vi "User Front Panel.vi"(8 "PanelCMDRef":refnum<vi>, 11 "PanelCluster":T6) -> ()   [LabVIEW 2019]
uses:
  <vilib>/Native 3D Graph/xcontrol/3DPC_SurfacePlot.xctl
  CoreModules/StationModule/StationData.ctl
panel:
  in  "Tab Control":enum32{"User", "Parameter"}(tab)
  out "PathPlot":refnum<class "Base Datatype.lvclass">[](xcontrol)
  in  "Test":bool
  in  "test123":bool
  in  "ID1":bool
  in  "ID2":bool
  in  "ID3":bool
  in  "ID4":bool
  in  "ID5":bool
  in  "ID6":bool
  in  "ID7":bool
  in  "ID8":bool
  in  "ID9":bool
  in  "ID10":bool
  in  "ID12":bool
  in  "ID11":bool
  in  "LensBuffer":T1
  in  "VcmBuffer":cluster{"1":bool, "2":bool, "3":bool, "4":bool}
  in  "testtray":T2
  out "appended path":path
  in  "FeedIn":T3
  in  "FeedOut":T4
  out "Image":T5(plugin-control)
  out "Waveform":waveform(dbl)[](graph)
  in  "CRDCMPT4Y":string
  in  "CRDCMPT4X":string
  in  "CRDCMPT4Org":string
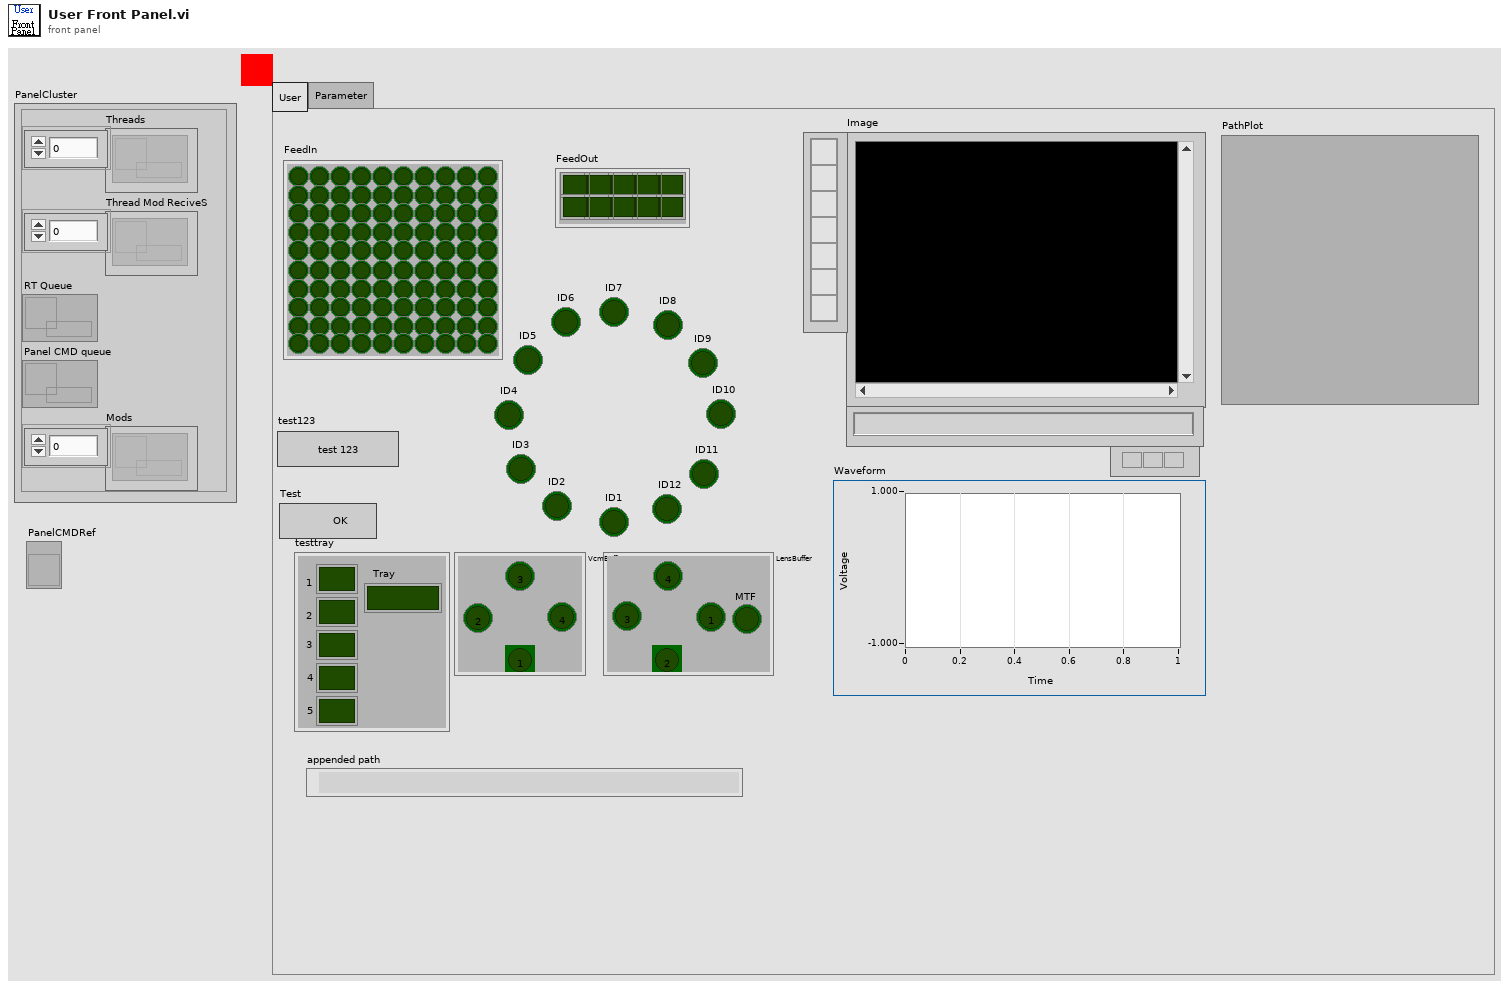
[diagram p1: front panel]
types:
  T1 = cluster{"MTF":bool, "1":bool, "2":bool, "3":bool, "4":bool}
  T2 = cluster{"Tray":bool, "1":bool, "2":bool, "3":bool, "4":bool, "5":bool}
  T3 = cluster{"1":bool, "2":bool, "3":bool, "4":bool, "5":bool, "6":bool, "7":bool, "8":bool, "9":bool, "10":bool, "1 2":bool, "2 2":bool, "3 2":bool, "4 2":bool, "5 2":bool, "6 2":bool, "7 2":bool, "8 2":bool, "9 2":bool, "10 2":bool, "1 3":bool, "2 3":bool, "3 3":bool, "4 3":bool, "5 3":bool, "6 3":bool, "7 3":bool, "8 3":bool, "9 3":bool, "10 3":bool, "1 4":bool, "2 4":bool, "3 4":bool, "4 4":bool, "5 4":bool, "6 4":bool, "7 4":bool, "8 4":bool, "9 4":bool, "10 4":bool, "1 5":bool, "2 5":bool, "3 5":bool, "4 5":bool, "5 5":bool, "6 5":bool, "7 5":bool, "8 5":bool, "9 5":bool, "10 5":bool, "1 6":bool, "2 6":bool, "3 6":bool, "4 6":bool, "5 6":bool, "6 6":bool, "7 6":bool, "8 6":bool, "9 6":bool, "10 6":bool, "1 7":bool, "2 7":bool, "3 7":bool, "4 7":bool, "5 7":bool, "6 7":bool, "7 7":bool, "8 7":bool, "9 7":bool, "10 7":bool, "1 8":bool, "2 8":bool, "3 8":bool, "4 8":bool, "5 8":bool, "6 8":bool, "7 8":bool, "8 8":bool, "9 8":bool, "10 8":bool, "1 9":bool, "2 9":bool, "3 9":bool, "4 9":bool, "5 9":bool, "6 9":bool, "7 9":bool, "8 9":bool, "9 9":bool, "10 9":bool, "1 10":bool, "2 10":bool, "3 10":bool, "4 10":bool, "5 10":bool, "6 10":bool, "7 10":bool, "8 10":bool, "9 10":bool, "10 10":bool}
  T4 = cluster{"1":bool, "2":bool, "3":bool, "4":bool, "5":bool, "1 2":bool, "2 2":bool, "3 2":bool, "4 2":bool, "5 2":bool}
  T5 = typedef "IMAQ Image.ctl" = refnum<image>
  T6 = cluster{"Threads":refnum<queue>[], "Thread Mod ReciveS":refnum<queue>[], "RT Queue":refnum<queue>, "Panel CMD queue":refnum<queue>, "Mods":refnum<queue>[]}
  T7 = typedef "StationData.ctl" = enum16{"ResetDefault", "SetStationOK", "SetStationNG", "UpdateIndicator", "GetData", "SetData", "StateShift", "Init", "SetStationON", "SetStationOFF", "BlinkingON", "BlinkingOFF"}
  T8 = enum16{"Init", "AddStation", "StateShift", "ResetDefault", "SetStationON", "SetStationOFF", "SetStationOK", "SetStationNG", "UpdateIndicator", "SetData", "GetData", "GetOnOff", "GetOkNg"}
  T9 = cluster{"Program":i32, "Prog Index":i32, "State Index":i32, "State":enum16{"Init", "Idle", "Auto Start", "Auto Running", "Step Start", "Step Running", "Suspend", "Restart", "Stop", "Reset"}}
  T10 = enum16{"Get", "UpdatePointS", "Init", "UpdateIndex", "GetCurrent&Index+1", "GetWithIndex", "ChkLast", "GetCurrent"}
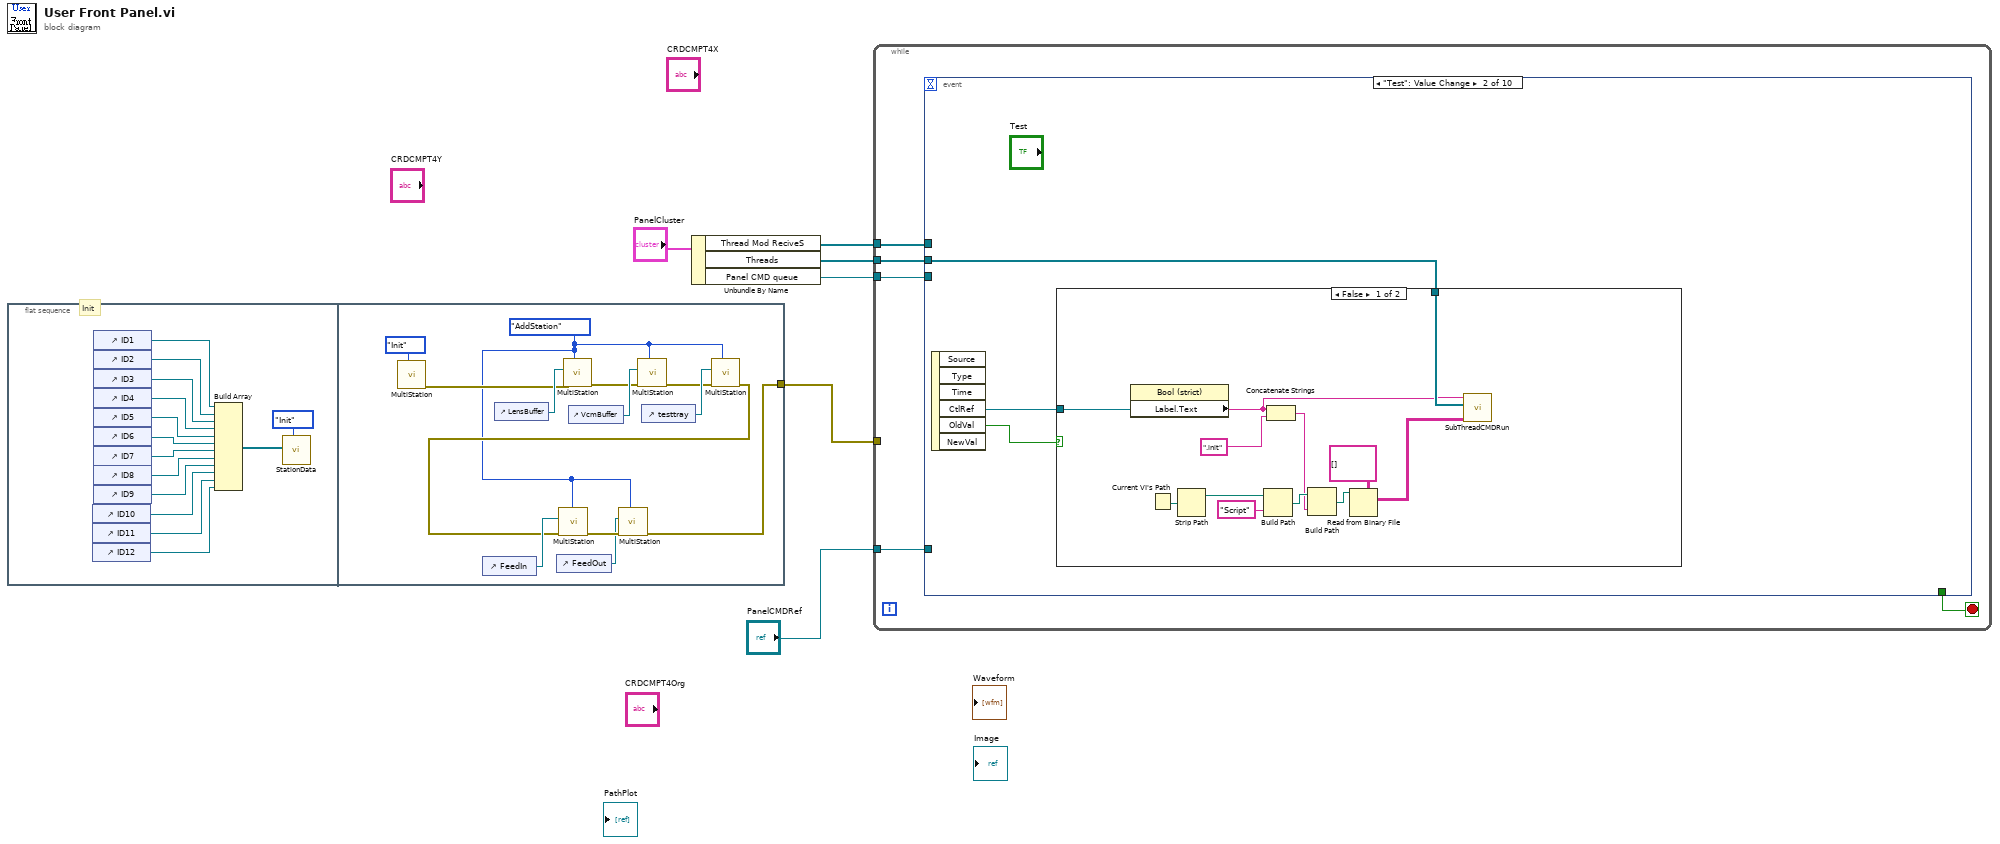
[diagram p0: block diagram]
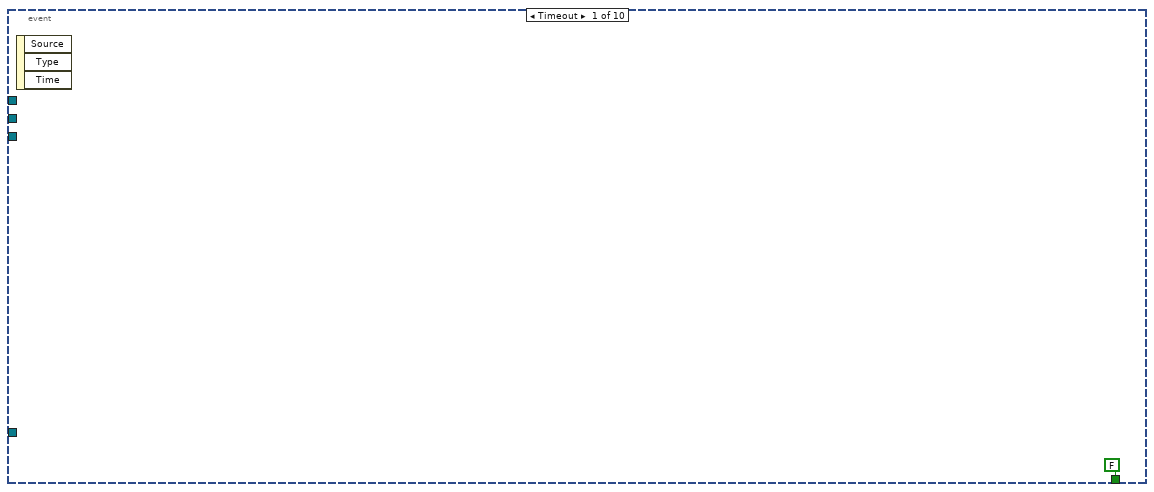
[diagram p2: hidden frame]
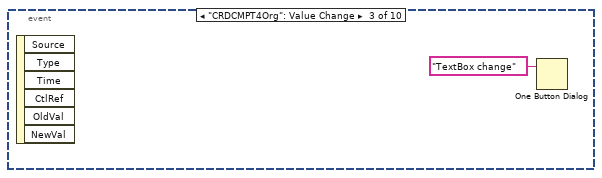
[diagram p4: hidden frame]
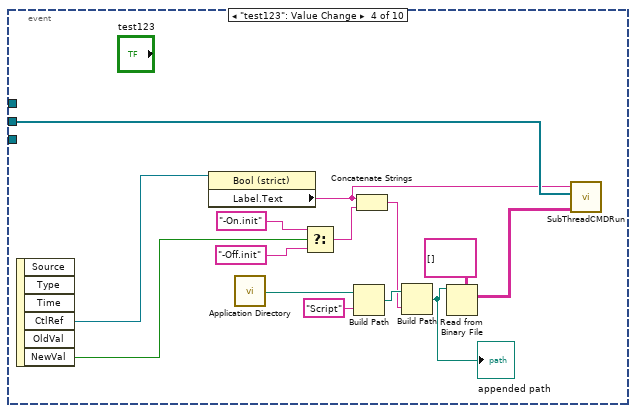
[diagram p5: hidden frame]
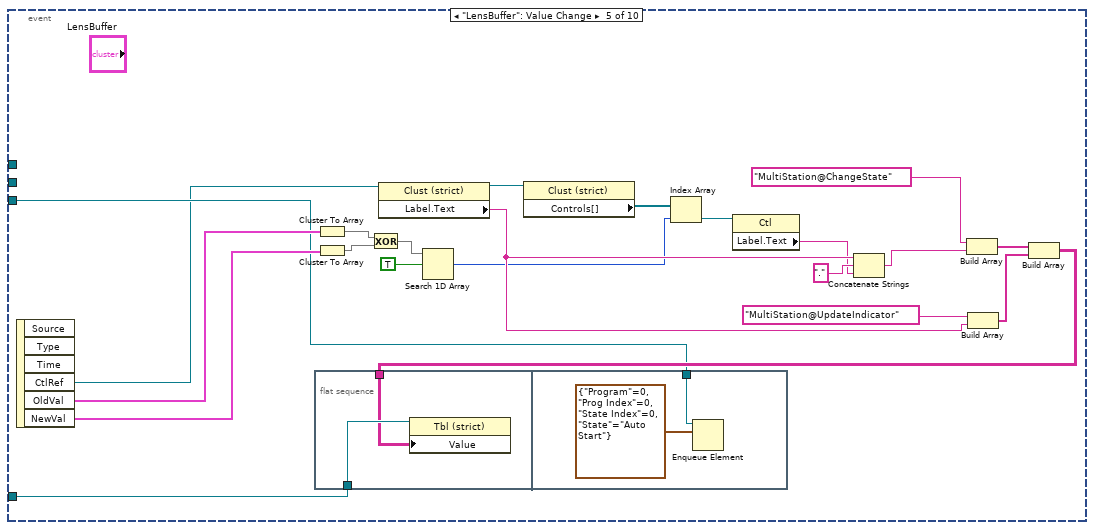
[diagram p6: hidden frame]
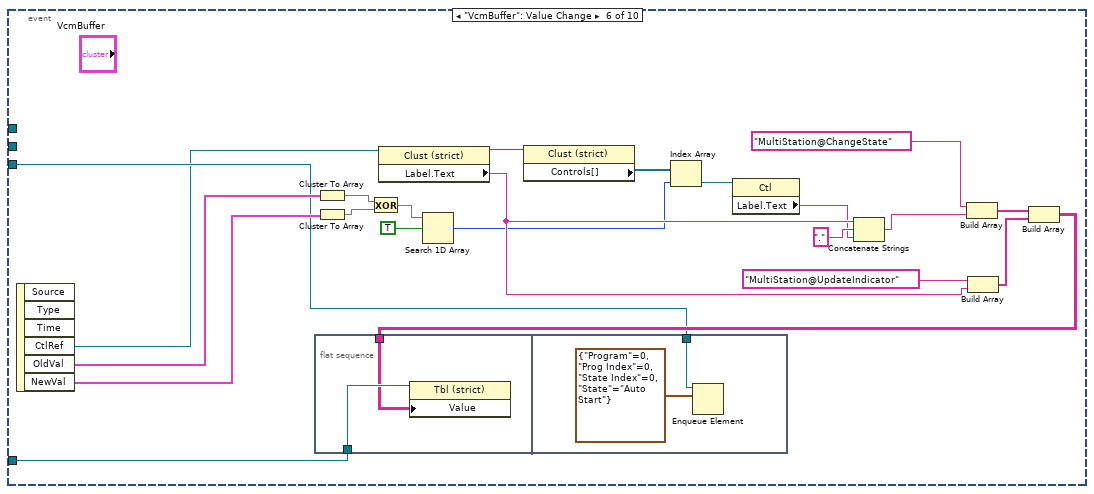
[diagram p7: hidden frame]
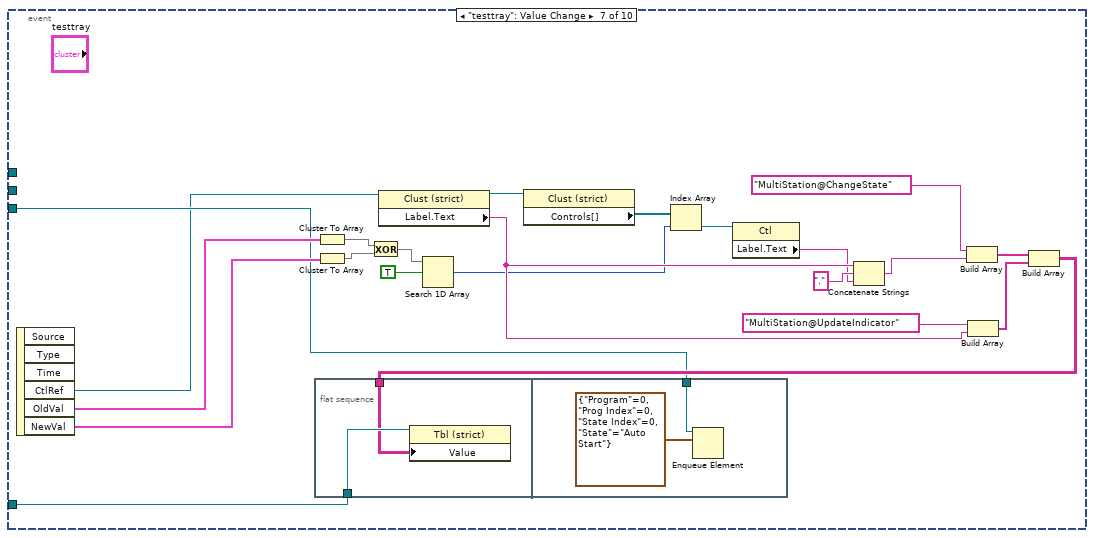
[diagram p8: hidden frame]
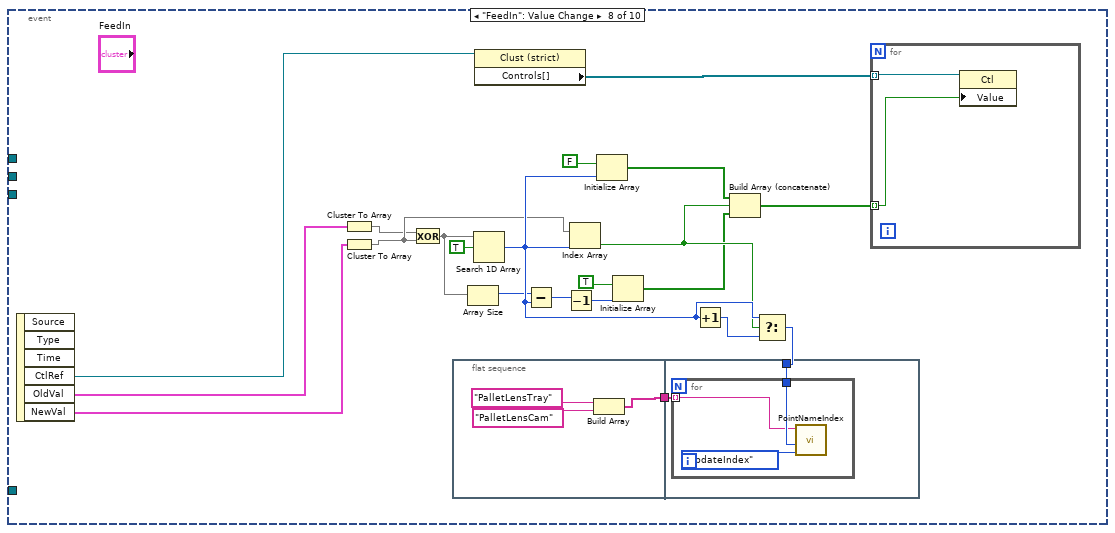
[diagram p9: hidden frame]
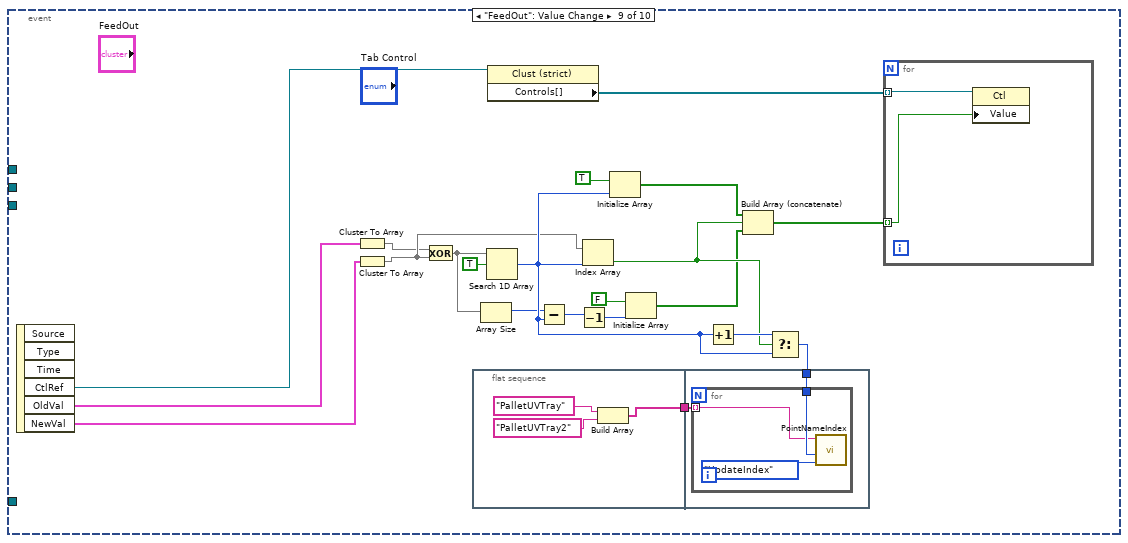
[diagram p10: hidden frame]
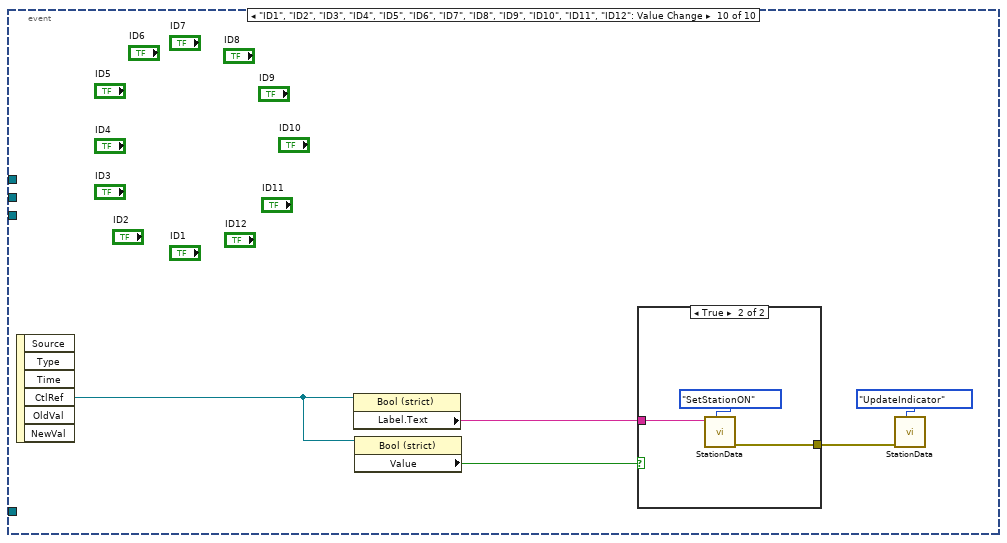
[diagram p11: hidden frame]
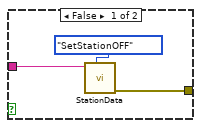
[diagram p12: hidden frame]
diagram:
  # "Init"
  n1 = flat-sequence {
    tunnel: [w22] -> w2
    frame #0 {
      n2 = control-ref of="ID10"() -> (w16:refnum<vi>)
      n3 = control-ref of="ID11"() -> (w17:refnum<vi>)
      n4 = control-ref of="ID12"() -> (w18:refnum<vi>)
      n5 = control-ref of="ID1"() -> (w7:refnum<vi>)
      n6 = control-ref of="ID2"() -> (w8:refnum<vi>)
      n7 = control-ref of="ID3"() -> (w9:refnum<vi>)
      n8 = control-ref of="ID4"() -> (w10:refnum<vi>)
      n9 = control-ref of="ID5"() -> (w11:refnum<vi>)
      n10 = control-ref of="ID6"() -> (w12:refnum<vi>)
      n11 = control-ref of="ID7"() -> (w13:refnum<vi>)
      n12 = control-ref of="ID8"() -> (w14:refnum<vi>)
      n13 = control-ref of="ID9"() -> (w15:refnum<vi>)
      n14 = Build Array(w7, w8, w9, w10, w11, w12, w13, w14, w15, w16, w17, w18) -> (w20:refnum<vi>[])
      n15 = call "StationData.vi"("CMD"=StationData."Init", "variant"=w20) -> ()  [unwired: 2 in, 8 out]
    }
    frame #1 {
      w23 = T8."AddStation" ("OP")
      n16 = call "MultiStation.vi"("OP"=T8."Init") -> ("error out"=w27:errorcluster)  [unwired: 6 in, 4 out]
      n17 = control-ref of="FeedIn"() -> (w26:refnum<vi>)
      n18 = control-ref of="LensBuffer"() -> (w33:refnum<vi>)
      n19 = control-ref of="FeedOut"() -> (w21:refnum<vi>)
      n20 = call "MultiStation.vi"("OP"=w23, "error in"=w27, "DataIn"=w33) -> ("error out"=w30:errorcluster)  [unwired: 4 in, 4 out]
      n21 = control-ref of="VcmBuffer"() -> (w32:refnum<vi>)
      n22 = call "MultiStation.vi"("OP"=w23, "error in"=w30, "DataIn"=w32) -> ("error out"=w29:errorcluster)  [unwired: 4 in, 4 out]
      n23 = control-ref of="testtray"() -> (w31:refnum<vi>)
      n24 = call "MultiStation.vi"("OP"=w23, "error in"=w29, "DataIn"=w31) -> ("error out"=w25:errorcluster)  [unwired: 4 in, 4 out]
      n25 = call "MultiStation.vi"("OP"=w23, "error in"=w25, "DataIn"=w26) -> ("error out"=w24:errorcluster)  [unwired: 4 in, 4 out]
      n26 = call "MultiStation.vi"("OP"=w23, "error in"=w24, "DataIn"=w21) -> ("error out"=w22:errorcluster)  [unwired: 4 in, 4 out]
    }
  }
  n27 = Unbundle By Name("PanelCluster") -> ("Thread Mod ReciveS"=w5:refnum<queue>[], "Threads"=w4:refnum<queue>[], "Panel CMD queue"=w3:refnum<queue>)
  n28 = while {
    tunnel: w5 -> [w36]
    tunnel: w4 -> [w37]
    tunnel: w3 -> [w35]
    tunnel: w2 -> [_]
    tunnel: "PanelCMDRef" -> [w34]
    stop <- w38 stop-if-true
    n29 = event shown="[1] \"Test\": Value Change" {
      selector: _ -> [_ _ _ _ _ _ _ _ _ _]
      dyn-events: _ -> [_ _ _ _ _ _ _ _ _ _]
      timeout: _ -> [_ _ _ _ _ _ _ _ _ _]
      tunnel: [FALSE _ _ _ _ _ _ _ _ _] -> w38
      tunnel: w37 -> [_ w42 _ w61 _ _ _ _ _ _]
      tunnel: w36 -> [_ _ _ _ _ _ _ _ _ _]
      tunnel: w35 -> [_ _ _ _ w72 w98 w124 _ _ _]
      tunnel: w34 -> [_ _ _ _ w70 w96 w122 _ _ _]
      event Timeout {
        n30 = event-data() -> ()  [unwired: 1 in, 3 out]
      }
      event "Test": Value Change {
        n31 = event-data() -> ("CtlRef"=w41:refnum<vi>, "OldVal"=w40:bool)  [unwired: 1 in, 4 out]
        n32 = case shown="False" w40 {
          tunnel: w42 -> [w54 _]
          tunnel: w41 -> [w53 _]
          frame False {
            n33 = property class="Bool (strict)"(reference=w53) -> ("Label.Text"=w43:string)  [unwired: 1 in, 2 out]
            n34 = Current VI's Path() -> (path=w47:path)
            n35 = Strip Path(path=w47) -> (stripped path=w46:path)  [unwired: 1 out]
            n36 = Build Path(base path=w46, name or relative path="Script") -> (appended path=w51:path)
            n37 = Concatenate Strings(w43, ".init" ("string")) -> (w50:string)
            n38 = Build Path(base path=w51, name or relative path=w50) -> (appended path=w49:path)
            n39 = Read from Binary File(5:string[][] [] ("Init Script"), 11:w49) -> (2:w45:string[][])  [unwired: 4 in, 3 out]
            n40 = call "SubThreadCMDRun.vi"("Command"=w45, "Threads"=w54, "SubThreadName"=w43) -> ()  [unwired: 8 in, 1 out]
          }
          frame True {
          }
        }
      }
      event "CRDCMPT4Org": Value Change {
        n41 = event-data() -> ()  [unwired: 1 in, 6 out]
        n42 = One Button Dialog(message="TextBox change") -> ()  [unwired: 1 in, 1 out]
      }
      event "test123": Value Change {
        n43 = event-data() -> ("CtlRef"=w60:refnum<vi>, "NewVal"=w59:bool)  [unwired: 1 in, 4 out]
        n44 = property class="Bool (strict)"(reference=w60) -> ("Label.Text"=w56:string)  [unwired: 1 in, 2 out]
        n45 = call <vilib>:"Application Directory.vi"() -> ("Application Directory"=w58:path)
        n46 = Select(t="-On.init", s=w59, f="-Off.init") -> (s? t:f=w65:string)
        n47 = Build Path(base path=w58, name or relative path="Script") -> (appended path=w68:path)
        n48 = Concatenate Strings(w56, w65) -> (w64:string)
        n49 = Build Path(base path=w68, name or relative path=w64) -> (appended path=w57:path)
        "appended path" <- w57
        n50 = Read from Binary File(5:string[][] [] ("Init Script"), 11:w57) -> (2:w62:string[][])  [unwired: 4 in, 3 out]
        n51 = call "SubThreadCMDRun.vi"("Command"=w62, "Threads"=w61, "SubThreadName"=w56) -> ()  [unwired: 8 in, 1 out]
      }
      event "LensBuffer": Value Change {
        n52 = event-data() -> ("CtlRef"=w71:refnum<vi>, "OldVal"=w74:T1, "NewVal"=w73:T1)  [unwired: 1 in, 3 out]
        n53 = flat-sequence {
          tunnel: w91 -> [w92]
          tunnel: w70 -> [w93]
          tunnel: w72 -> [w94]
          frame #0 {
            n54 = property class="Tbl (strict)"(reference=w93, "Value"=w92) -> ()  [unwired: 1 in, 2 out]
          }
          frame #1 {
            n55 = Enqueue Element(queue=w94, element=T9 {"Program"=0, "Prog Index"=0, "State Index"=0, "State"=enum."Auto Start"}) -> ()  [unwired: 1 in, 4 out]
          }
        }
        n56 = Cluster To Array(cluster=w74) -> (array=w75:bool[])
        n57 = Cluster To Array(cluster=w73) -> (array=w76:bool[])
        n58 = Exclusive Or(1:w76, 2:w75) -> (0:w77:bool[])
        n59 = property class="Clust (strict)"(reference=w71) -> (reference out=w79:refnum<vi>, "Label.Text"=w89:string)  [unwired: 1 in, 1 out]
        n60 = Search 1D Array(1D array=w77, element=TRUE) -> (index of element=w81:i32)  [unwired: 1 in]
        n61 = property class="Clust (strict)"(reference=w79) -> ("Controls[]"=w80:refnum<vi>[])  [unwired: 1 in, 2 out]
        n62 = Index Array(array=w80, index=w81) -> (element=w82:refnum<vi>)
        n63 = property class="Ctl"(reference=w82) -> ("Label.Text"=w83:string)  [unwired: 1 in, 2 out]
        n64 = Concatenate Strings(w89, "." ("string"), w83) -> (w86:string)
        n65 = Build Array("MultiStation@ChangeState", w86) -> (w87:string[])
        n66 = Build Array("MultiStation@UpdateIndicator", w89) -> (w90:string[])
        n67 = Build Array(w87, w90) -> (w91:string[][])
      }
      event "VcmBuffer": Value Change {
        n68 = event-data() -> ("CtlRef"=w97:refnum<vi>, "OldVal"=w100:cluster{"1":bool, "2":bool, "3":bool, "4":bool}, "NewVal"=w99:cluster{"1":bool, "2":bool, "3":bool, "4":bool})  [unwired: 1 in, 3 out]
        n69 = flat-sequence {
          tunnel: w117 -> [w118]
          tunnel: w96 -> [w119]
          tunnel: w98 -> [w120]
          frame #0 {
            n70 = property class="Tbl (strict)"(reference=w119, "Value"=w118) -> ()  [unwired: 1 in, 2 out]
          }
          frame #1 {
            n71 = Enqueue Element(queue=w120, element=T9 {"Program"=0, "Prog Index"=0, "State Index"=0, "State"=enum."Auto Start"}) -> ()  [unwired: 1 in, 4 out]
          }
        }
        n72 = Cluster To Array(cluster=w100) -> (array=w101:bool[])
        n73 = Cluster To Array(cluster=w99) -> (array=w102:bool[])
        n74 = Exclusive Or(1:w102, 2:w101) -> (0:w103:bool[])
        n75 = property class="Clust (strict)"(reference=w97) -> (reference out=w105:refnum<vi>, "Label.Text"=w115:string)  [unwired: 1 in, 1 out]
        n76 = Search 1D Array(1D array=w103, element=TRUE) -> (index of element=w107:i32)  [unwired: 1 in]
        n77 = property class="Clust (strict)"(reference=w105) -> ("Controls[]"=w106:refnum<vi>[])  [unwired: 1 in, 2 out]
        n78 = Index Array(array=w106, index=w107) -> (element=w108:refnum<vi>)
        n79 = property class="Ctl"(reference=w108) -> ("Label.Text"=w109:string)  [unwired: 1 in, 2 out]
        n80 = Concatenate Strings(w115, "." ("string"), w109) -> (w112:string)
        n81 = Build Array("MultiStation@ChangeState", w112) -> (w113:string[])
        n82 = Build Array("MultiStation@UpdateIndicator", w115) -> (w116:string[])
        n83 = Build Array(w113, w116) -> (w117:string[][])
      }
      event "testtray": Value Change {
        n84 = event-data() -> ("CtlRef"=w123:refnum<vi>, "OldVal"=w126:T2, "NewVal"=w125:T2)  [unwired: 1 in, 3 out]
        n85 = flat-sequence {
          tunnel: w143 -> [w144]
          tunnel: w122 -> [w145]
          tunnel: w124 -> [w146]
          frame #0 {
            n86 = property class="Tbl (strict)"(reference=w145, "Value"=w144) -> ()  [unwired: 1 in, 2 out]
          }
          frame #1 {
            n87 = Enqueue Element(queue=w146, element=T9 {"Program"=0, "Prog Index"=0, "State Index"=0, "State"=enum."Auto Start"}) -> ()  [unwired: 1 in, 4 out]
          }
        }
        n88 = Cluster To Array(cluster=w126) -> (array=w127:bool[])
        n89 = Cluster To Array(cluster=w125) -> (array=w128:bool[])
        n90 = Exclusive Or(1:w128, 2:w127) -> (0:w129:bool[])
        n91 = property class="Clust (strict)"(reference=w123) -> (reference out=w131:refnum<vi>, "Label.Text"=w141:string)  [unwired: 1 in, 1 out]
        n92 = Search 1D Array(1D array=w129, element=TRUE) -> (index of element=w133:i32)  [unwired: 1 in]
        n93 = property class="Clust (strict)"(reference=w131) -> ("Controls[]"=w132:refnum<vi>[])  [unwired: 1 in, 2 out]
        n94 = Index Array(array=w132, index=w133) -> (element=w134:refnum<vi>)
        n95 = property class="Ctl"(reference=w134) -> ("Label.Text"=w135:string)  [unwired: 1 in, 2 out]
        n96 = Concatenate Strings(w141, "." ("string"), w135) -> (w138:string)
        n97 = Build Array("MultiStation@ChangeState", w138) -> (w139:string[])
        n98 = Build Array("MultiStation@UpdateIndicator", w141) -> (w142:string[])
        n99 = Build Array(w139, w142) -> (w143:string[][])
      }
      event "FeedIn": Value Change {
        n100 = event-data() -> ("CtlRef"=w150:refnum<vi>, "OldVal"=w149:T3, "NewVal"=w148:T3)  [unwired: 1 in, 3 out]
        n101 = Cluster To Array(cluster=w149) -> (array=w151:bool[])
        n102 = Cluster To Array(cluster=w148) -> (array=w161:bool[])
        n103 = Exclusive Or(1:w161, 2:w151) -> (0:w154:bool[])
        n104 = flat-sequence {
          tunnel: [w169] -> w168
          tunnel: w165 -> [w173]
          tunnel: w168 -> [w172]
          frame #0 {
            n105 = Build Array("PalletLensTray", "PalletLensCam") -> (w169:string[])
          }
          frame #1 {
            n106 = for {
              tunnel: w173 -> [w176]
              tunnel: w172 -> [w175] mode=indexing
              n107 = call "PointNameIndex.vi"("OP"=T10."UpdateIndex", "PathIndexIn"=w176, "PointName"=w175) -> ()  [unwired: 3 in, 6 out]
            }
          }
        }
        n108 = Array Size(array=w154) -> (size(s)=w155:i32)
        n109 = Search 1D Array(1D array=w154, element=TRUE) -> (index of element=w167:i32)  [unwired: 1 in]
        n110 = property class="Clust (strict)"(reference=w150) -> ("Controls[]"=w162:refnum<vi>[])  [unwired: 1 in, 2 out]
        n111 = Subtract(x=w155, y=w167) -> (x-y=w159:i32)
        n112 = Decrement(x=w159) -> (x-1=w160:i32)
        n113 = Index Array(array=w161, index=w167) -> (element=w164:bool)
        n114 = Initialize Array(FALSE ("element"), w167) -> (w157:bool[])
        n115 = Initialize Array(TRUE ("element"), w160) -> (w158:bool[])
        n116 = Increment(x=w167) -> (x+1=w166:i32)
        n117 = Build Array (concatenate)(w157, w164, w158) -> (w163:bool[])
        n118 = Select(t=w167, s=w164, f=w166) -> (s? t:f=w165:i32)
        n119 = for {
          tunnel: w162 -> [w178] mode=indexing
          tunnel: w163 -> [w177] mode=indexing
          n120 = property class="Ctl"(reference=w178, "Value"=w177) -> ()  [unwired: 1 in, 2 out]
        }
      }
      event "FeedOut": Value Change {
        n121 = event-data() -> ("CtlRef"=w181:refnum<vi>, "OldVal"=w180:T4, "NewVal"=w179:T4)  [unwired: 1 in, 3 out]
        n122 = Cluster To Array(cluster=w180) -> (array=w182:bool[])
        n123 = Cluster To Array(cluster=w179) -> (array=w192:bool[])
        n124 = Exclusive Or(1:w192, 2:w182) -> (0:w185:bool[])
        n125 = flat-sequence {
          tunnel: [w200] -> w199
          tunnel: w196 -> [w204]
          tunnel: w199 -> [w203]
          frame #0 {
            n126 = Build Array("PalletUVTray", "PalletUVTray2") -> (w200:string[])
          }
          frame #1 {
            n127 = for {
              tunnel: w204 -> [w207]
              tunnel: w203 -> [w206] mode=indexing
              n128 = call "PointNameIndex.vi"("OP"=T10."UpdateIndex", "PathIndexIn"=w207, "PointName"=w206) -> ()  [unwired: 3 in, 6 out]
            }
          }
        }
        n129 = Array Size(array=w185) -> (size(s)=w186:i32)
        n130 = Search 1D Array(1D array=w185, element=TRUE) -> (index of element=w198:i32)  [unwired: 1 in]
        n131 = property class="Clust (strict)"(reference=w181) -> ("Controls[]"=w193:refnum<vi>[])  [unwired: 1 in, 2 out]
        n132 = Subtract(x=w186, y=w198) -> (x-y=w190:i32)
        n133 = Decrement(x=w190) -> (x-1=w191:i32)
        n134 = Index Array(array=w192, index=w198) -> (element=w195:bool)
        n135 = Initialize Array(TRUE ("element"), w198) -> (w188:bool[])
        n136 = Initialize Array(FALSE ("element"), w191) -> (w189:bool[])
        n137 = Increment(x=w198) -> (x+1=w197:i32)
        n138 = Build Array (concatenate)(w188, w195, w189) -> (w194:bool[])
        n139 = Select(t=w197, s=w195, f=w198) -> (s? t:f=w196:i32)
        n140 = for {
          tunnel: w193 -> [w209] mode=indexing
          tunnel: w194 -> [w208] mode=indexing
          n141 = property class="Ctl"(reference=w209, "Value"=w208) -> ()  [unwired: 1 in, 2 out]
        }
      }
      event "ID1", "ID2", "ID3", "ID4", "ID5", "ID6", "ID7", "ID8", "ID9", "ID10", "ID11", "ID12": Value Change {
        n142 = event-data() -> ("CtlRef"=w210:refnum<vi>)  [unwired: 1 in, 5 out]
        n143 = property class="Bool (strict)"(reference=w210) -> ("Label.Text"=w212:string)  [unwired: 1 in, 2 out]
        n144 = property class="Bool (strict)"(reference=w210) -> ("Value"=w211:bool)  [unwired: 1 in, 2 out]
        n145 = case shown="True" w211 {
          tunnel: w212 -> [w216 w219]
          tunnel: [w215 w218] -> w214
          frame False {
            n146 = call "StationData.vi"("CMD"=StationData."SetStationOFF", "StationID"=w216) -> ("error out"=w215:errorcluster)  [unwired: 2 in, 7 out]
          }
          frame True {
            n147 = call "StationData.vi"("CMD"=StationData."SetStationON", "StationID"=w219) -> ("error out"=w218:errorcluster)  [unwired: 2 in, 7 out]
          }
        }
        n148 = call "StationData.vi"("CMD"=StationData."UpdateIndicator", "error in"=w214) -> ()  [unwired: 2 in, 8 out]
      }
    }
  }
